vi "Send Command.vi"(8 "text":string, 9 "cmd":T2=enum."move", 10 "Type":T1, 11 "Coords":T3) -> ()   [LabVIEW 2020, in "Graph Extensions.lvlib"]
doc: "This function is needed for sending commands (events) from the graph UI to the marker draw service. \n\nNeeded events and commands are:\n<b>Mouse Move</b> (only coordinates are needed as an input)\n<b>Mouse Down</b> (a code block is needed for down events, where this cmd is included in it, so should not be used on its own for down events)\n<b>Mouse Up</b> a code block is needed for up events, where this cmd is included in it, so should not be used on its own for up events)\n<b>Exit</b> (no inputs are requred)\nExit"
uses:
  Graph Extensions.lvlib
  <vilib>/Utility/miscctls.llb/LVPoint32TypeDef.ctl
  controls/commands.ctl
  controls/markerType.ctl
  controls/GraphExt-Cmds.ctl
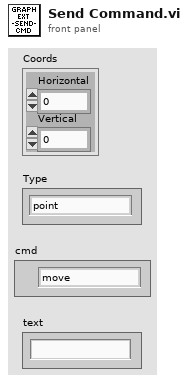
[diagram p1: front panel]
types:
  T1 = typedef "Graph Extensions.lvlib/markerType.ctl" = enum16{"point", "arrow", "horiz", "vert", "vert range", "horiz range", "box"}
  T2 = typedef "Graph Extensions.lvlib/commands.ctl" = enum16{"up", "options", "click", "move", "type", "redraw", "edited", "exit"}
  T3 = typedef "LVPoint32TypeDef.ctl" = cluster{"Horizontal":dbl, "Vertical":dbl}
  T4 = typedef "Graph Extensions.lvlib/GraphExt-Cmds.ctl" = cluster{"cmd":T2, "Type":T1, "Coords":T3, "text":string}
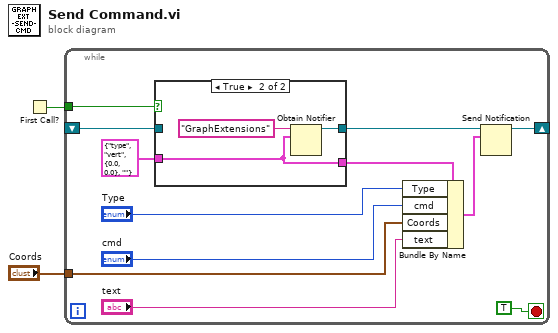
[diagram p0: block diagram]
diagram:
  n1 = First Call?() -> (First Call?: T/F=w1:bool)
  n2 = while {
    tunnel: "Coords" -> [w10]
    shift-right: [w8] -> _
    shift-left: _ -> [w7]
    tunnel: w1 -> [w9]
    stop <- TRUE stop-if-true
    n3 = case shown="True" w9 {
      tunnel: [w15 w17] -> w14
      tunnel: [w16 w19] -> w13
      tunnel: w7 -> [w16 _]
      tunnel: T4 {"cmd"=enum."type", "Type"=enum."vert", "Coords"={"Horizontal"=0.0, "Vertical"=0.0}, "text"=""} -> [w15 w17]
      frame False {
      }
      frame True {
        n4 = Obtain Notifier(name (unnamed)="GraphExtensions", notification data type=w17) -> (notifier out=w19:refnum<notifier>)  [unwired: 2 in, 2 out]
      }
    }
    n5 = Bundle By Name(cluster=w14, "Type"="Type", "cmd"="cmd", "Coords"=w10, "text"="text") -> (w11:T4)
    n6 = Send Notification(notification=w11, notifier=w13) -> (notifier out=w8:refnum<notifier>)  [unwired: 1 in, 1 out]
  }
